vi "Save Collimation Data.vi"(5 "Data":string[](array[string]), 7 "Item":string[](array[string]), 8 "Error In":errorcluster, 11 "路径":string) -> (0 "error out":errorcluster caption="错误输出")   [LabVIEW 2018]
uses:
  <vilib>/Utility/file.llb/Write Delimited Spreadsheet (string).vi
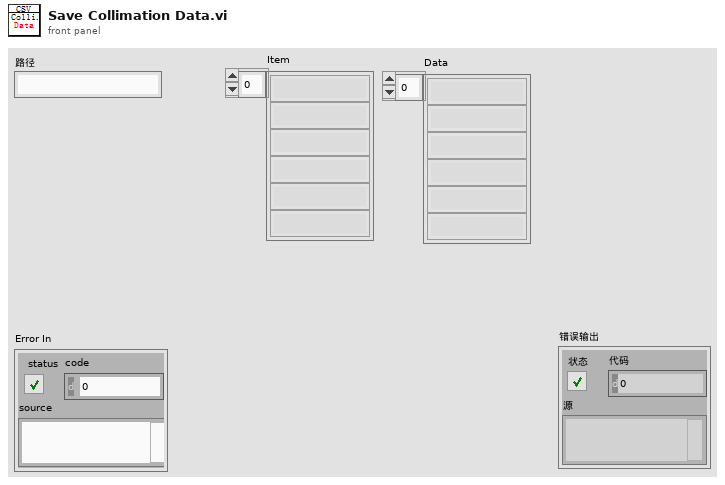
[diagram p1: front panel]
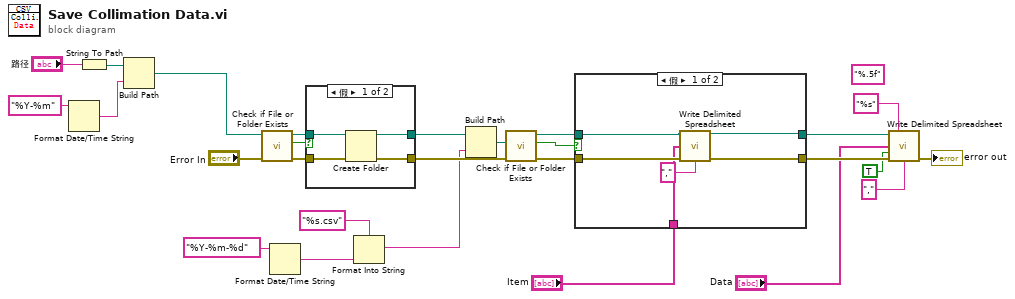
[diagram p0: block diagram]
diagram:
  (unwired) "%.5f" ("format (%s)")
  n1 = Format Date/Time String(time format string (%c)="%Y-%m") -> (date/time string=w14:string)  [unwired: 2 in]
  n2 = String To Path(string="路径") -> (path=w15:path)
  n3 = Build Path(base path=w15, name or relative path=w14) -> (appended path=w4:path)
  n4 = call <vilib>:"Check if File or Folder Exists.vi"("error in (no error)"="Error In", "path"=w4) -> ("error out"=w25:errorcluster, "file or folder exists?"=w26:bool, "dup path"=w23:path)  [unwired: 7 in]
  n5 = Format Date/Time String(time format string (%c)="%Y-%m-%d") -> (date/time string=w2:string)  [unwired: 2 in]
  n6 = case shown="假" w26 {
    tunnel: w25 -> [w30 w32]
    tunnel: w23 -> [w31 w33]
    tunnel: [w29 w33] -> w20
    tunnel: [w28 w32] -> w22
    frame False {
      n7 = Create Folder(path (use dialog)=w31, error in=w30) -> (created path=w29:path, error out=w28:errorcluster)  [unwired: 1 in, 1 out]
    }
    frame True {
    }
  }
  n8 = Format Into String(format string="%s.csv" ("格式字符串"), w2) -> (resulting string=w12:string)  [unwired: 2 in, 1 out]
  n9 = Build Path(base path=w20, name or relative path=w12) -> (appended path=w21:path)
  n10 = call <vilib>:"Check if File or Folder Exists.vi"("error in (no error)"=w22, "path"=w21) -> ("error out"=w17:errorcluster, "file or folder exists?"=w19:bool, "dup path"=w18:path)  [unwired: 7 in]
  n11 = case shown="假" w19 {
    tunnel: w18 -> [w39 w41]
    tunnel: w17 -> [w37 w40]
    tunnel: [w38 w41] -> w11
    tunnel: [w36 w40] -> w10
    tunnel: "Item" -> [w35 _]
    frame False {
      n12 = call-poly <vilib>:"Write Delimited Spreadsheet.vi"("file path (dialog if empty)"=w39, "1D data"=w35, "error in (no error)"=w37, "delimiter (\\t)"="," ("delimiter (\\t)")) -> ("new file path (Not A Path if cancelled)"=w38:path, "error out"=w36:errorcluster)  [unwired: 10 in]
    }
    frame True {
    }
  }
  n13 = call-poly <vilib>:"Write Delimited Spreadsheet.vi"("file path (dialog if empty)"=w11, "format (%s)"="%s", "1D data"="Data", "append to file? (new file:F)"=TRUE, "error in (no error)"=w10, "delimiter (\\t)"="," ("delimiter (\\t)")) -> ("error out"=→"error out":errorcluster)  [unwired: 8 in, 1 out]
